vi "FT10_M4X Simulate Read.vi"() -> (0 "Analysis Cluster Array - Current":T2[](array[typedef]), 1 "seconds since 1Jan1904":timestamp, 2 "Log Waveform Cluster - Current":T1, 3 "Simulated Log Analysis Cluster  - Current":T2, 5 "Simulated Waveform Array - Current":T1[](array[typedef]))   [LabVIEW 2015]
doc: "Simulate random values for waveforms and analysis clusters.\n\nIntended for debugging purposes."
uses:
  Controls/Control_Log Analysis Cluster - Current.ctl
  Controls/Control_Log Waveform Cluster - Current.ctl
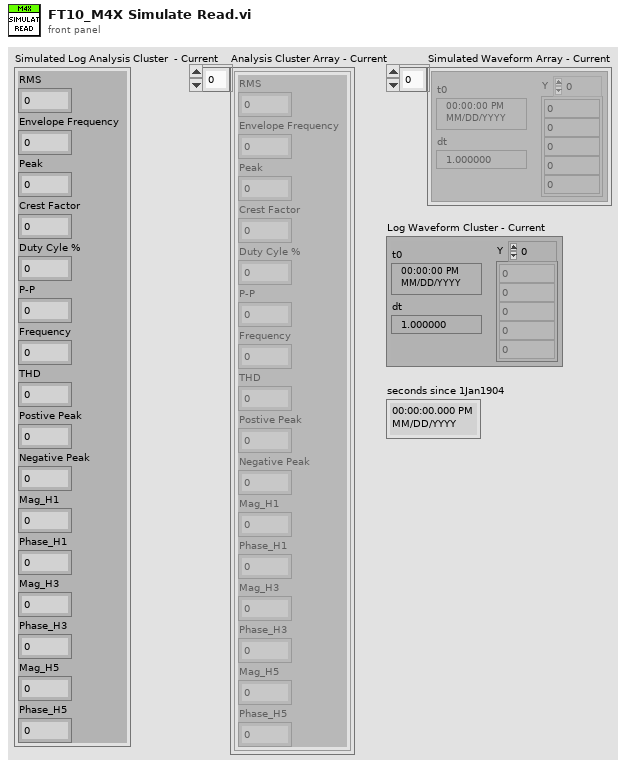
[diagram p1: front panel]
types:
  T1 = typedef "Control_Log Waveform Cluster - Current.ctl" = waveform(dbl)
  T2 = typedef "Control_Log Analysis Cluster - Current.ctl" = cluster{"RMS":dbl, "Envelope Frequency":dbl, "Peak":dbl, "Crest Factor":dbl, "Duty Cyle %":dbl, "P-P":dbl, "Frequency":dbl, "THD":dbl, "Postive Peak":dbl, "Negative Peak":dbl, "Mag_H1":dbl, "Phase_H1":dbl, "Mag_H3":dbl, "Phase_H3":dbl, "Mag_H5":dbl, "Phase_H5":dbl}
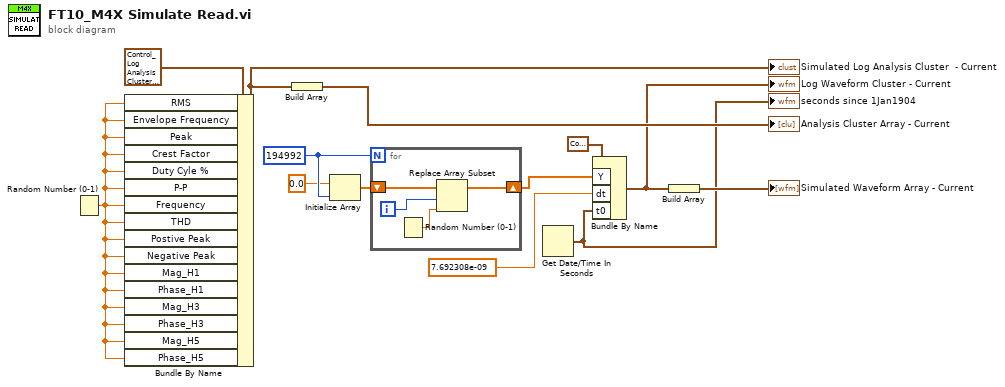
[diagram p0: block diagram]
diagram:
  w2 = 194992 ("memsize")
  n1 = Random Number (0-1)() -> (number: 0 to 1=w10:dbl)
  n2 = Bundle By Name(cluster=T2 {"RMS"=0.0, "Envelope Frequency"=0.0, "Peak"=0.0, "Crest Factor"=0.0, "Duty Cyle %"=0.0, "P-P"=0.0, "Frequency"=0.0, "THD"=0.0, "Postive Peak"=0.0, "Negative Peak"=0.0, "Mag_H1"=0.0, "Phase_H1"=0.0, "Mag_H3"=0.0, "Phase_H3"=0.0, "Mag_H5"=0.0, "Phase_H5"=0.0} ("Log Analysis Cluster"), "RMS"=w10, "Envelope Frequency"=w10, "Peak"=w10, "Crest Factor"=w10, "Duty Cyle %"=w10, "P-P"=w10, "Frequency"=w10, "THD"=w10, "Postive Peak"=w10, "Negative Peak"=w10, "Mag_H1"=w10, "Phase_H1"=w10, "Mag_H3"=w10, "Phase_H3"=w10, "Mag_H5"=w10, "Phase_H5"=w10) -> (w13:T2)
  "Simulated Log Analysis Cluster  - Current" <- w13
  n3 = Build Array(w13) -> (→"Analysis Cluster Array - Current":T2[])
  n4 = Initialize Array(0.0 ("element"), w2) -> (w3:dbl[])
  n5 = for {
    N: w2 -> [_]
    shift-right: [w16] -> w4
    shift-left: w3 -> [w17]
    i -> [w15]
    n6 = Random Number (0-1)() -> (number: 0 to 1=w14:dbl)
    n7 = Replace Array Subset(array=w17, new element=w14, index=w15) -> (w16:dbl[])
  }
  n8 = Get Date/Time In Seconds() -> (seconds since 1Jan1904=w7:timestamp)
  "seconds since 1Jan1904" <- w7
  n9 = Bundle By Name(cluster=T1 {"t0"=timestamp(0 s since 1904-01-01), "dt"=1.0, "Y"=[]} ("Log Waveform Cluster"), "Y"=w4, "dt"=7.692308e-09, "t0"=w7) -> (w8:T1)
  "Log Waveform Cluster - Current" <- w8
  n10 = Build Array(w8) -> (→"Simulated Waveform Array - Current":T1[])
